vi "NCC Local Sums.vi"(0 "Input Array":dbl[][](array[numeric]), 9 "Row Pad":i32, 11 "Col Pad":i32) -> (8 "Local Sum":dbl[][](array[numeric]))   [LabVIEW 2020]
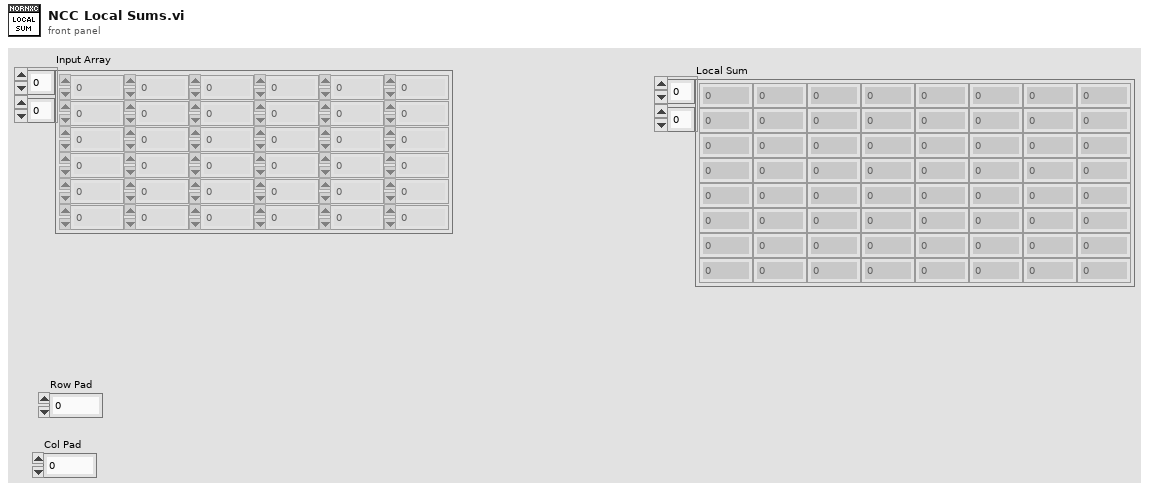
[diagram p1: front panel]
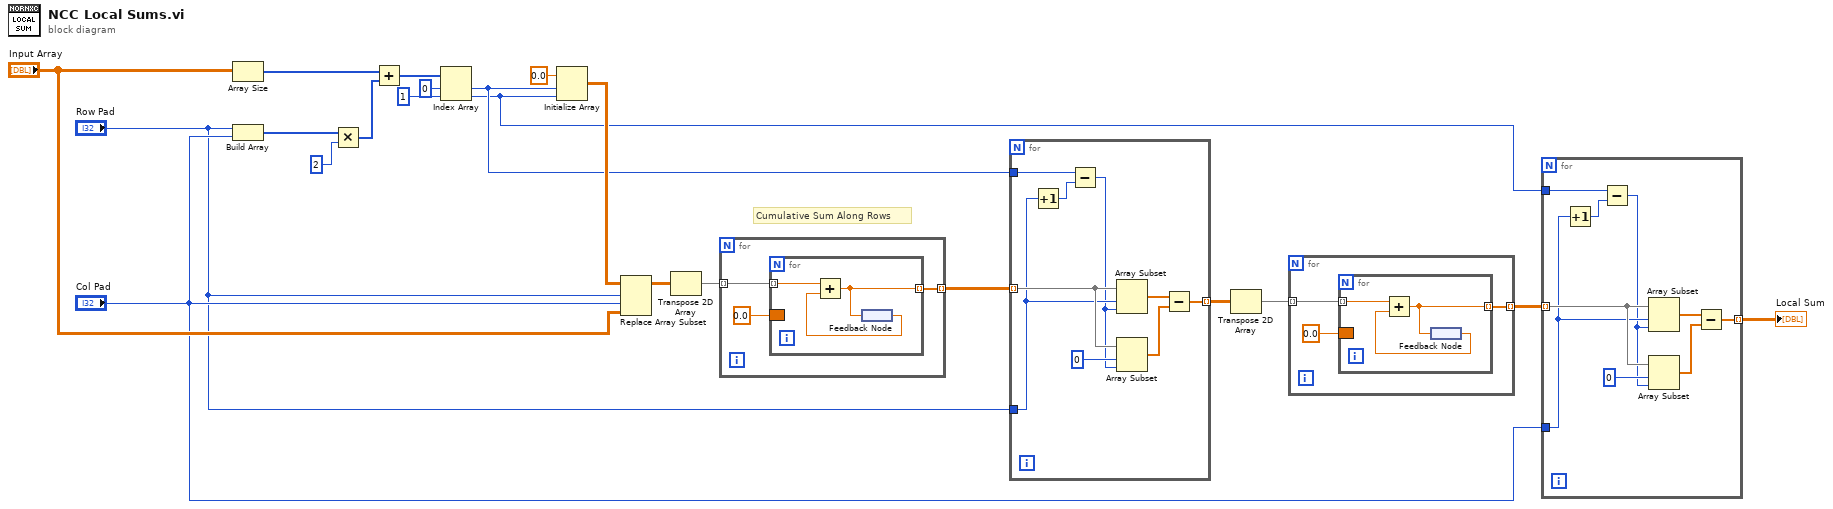
[diagram p0: block diagram]
diagram:
  # "Cumulative Sum Along Rows"
  n1 = Array Size(array="Input Array") -> (size(s)=w21:i32[])
  n2 = Build Array("Row Pad", "Col Pad") -> (w20:i32[])
  n3 = Multiply(x=w20, y=2) -> (x*y=w18:i32[])
  n4 = Add(x=w21, y=w18) -> (x+y=w16:i32[])
  n5 = Index Array(array=w16, index #1=0 ("index"), index #2=1 ("index")) -> (element #1=w8:i32, element #2=w3:i32)
  n6 = Initialize Array(0.0 ("element"), w8, w3) -> (w13:dbl[][])
  n7 = Replace Array Subset(array=w13, new element="Input Array", index (row)="Row Pad", index (col)="Col Pad") -> (w11:dbl[][])
  n8 = Transpose 2D Array(2D array=w11) -> (transposed array=w10:dbl[][])
  n9 = for {
    tunnel: w10 -> [w24] mode=indexing
    tunnel: [w23] -> w9 mode=indexing
    n10 = for {
      tunnel: w24 -> [w27] mode=indexing
      border: 0.0 -> [_]
      tunnel: [w25] -> w23 mode=indexing
      n11 = feedback #1() -> (w26:dbl)
      n12 = Add(x=w27, y=w26) -> (x+y=w25:dbl)
      n13 = feedback-in #1(w25) -> ()
    }
  }
  n14 = for {
    tunnel: w9 -> [w34] mode=indexing
    tunnel: "Row Pad" -> [w31]
    tunnel: w8 -> [w32]
    tunnel: [w28] -> w7 mode=indexing
    n15 = Increment(x=w31) -> (x+1=w30:i32)
    n16 = Subtract(x=w32, y=w30) -> (x-y=w29:i32)
    n17 = Array Subset(array=w34, index=w31, length=w29) -> (w36:dbl[])
    n18 = Array Subset(array=w34, index=0, length=w29) -> (w35:dbl[])
    n19 = Subtract(x=w36, y=w35) -> (x-y=w28:dbl[])
  }
  n20 = Transpose 2D Array(2D array=w7) -> (transposed array=w6:dbl[][])
  n21 = for {
    tunnel: w6 -> [w39] mode=indexing
    tunnel: [w38] -> w5 mode=indexing
    n22 = for {
      tunnel: w39 -> [w42] mode=indexing
      border: 0.0 -> [_]
      tunnel: [w40] -> w38 mode=indexing
      n23 = feedback #2() -> (w41:dbl)
      n24 = Add(x=w42, y=w41) -> (x+y=w40:dbl)
      n25 = feedback-in #2(w40) -> ()
    }
  }
  n26 = for {
    tunnel: w5 -> [w49] mode=indexing
    tunnel: "Col Pad" -> [w46]
    tunnel: w3 -> [w47]
    tunnel: [w43] -> w4 mode=indexing
    n27 = Increment(x=w46) -> (x+1=w45:i32)
    n28 = Subtract(x=w47, y=w45) -> (x-y=w44:i32)
    n29 = Array Subset(array=w49, index=w46, length=w44) -> (w51:dbl[])
    n30 = Array Subset(array=w49, index=0, length=w44) -> (w50:dbl[])
    n31 = Subtract(x=w51, y=w50) -> (x-y=w43:dbl[])
  }
  "Local Sum" <- w4
